vi "Example - Simple Move.vi"() -> ()   [LabVIEW 2017]
uses:
  SmartMotor_class/SmartMotor.lvclass
panel:
  in  "Start Motor 3":bool
  in  "Stop Motor 3":bool
  in  "Reset Motor Faults":bool
  in  "Start Motor 2":bool
  in  "Stop Motor 2":bool
  in  "SmartMotor Chain VISA Resource":refnum<visa-resource-name>="COM12"
  in  "Number of Motors In Motor Chain":i32=6 min=0 max=10 step=1
  in  "Start Motor":bool
  in  "Stop Motor":bool
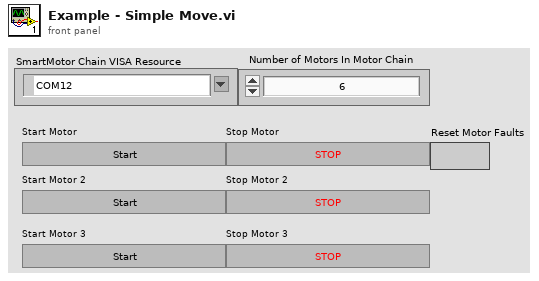
[diagram p1: front panel]
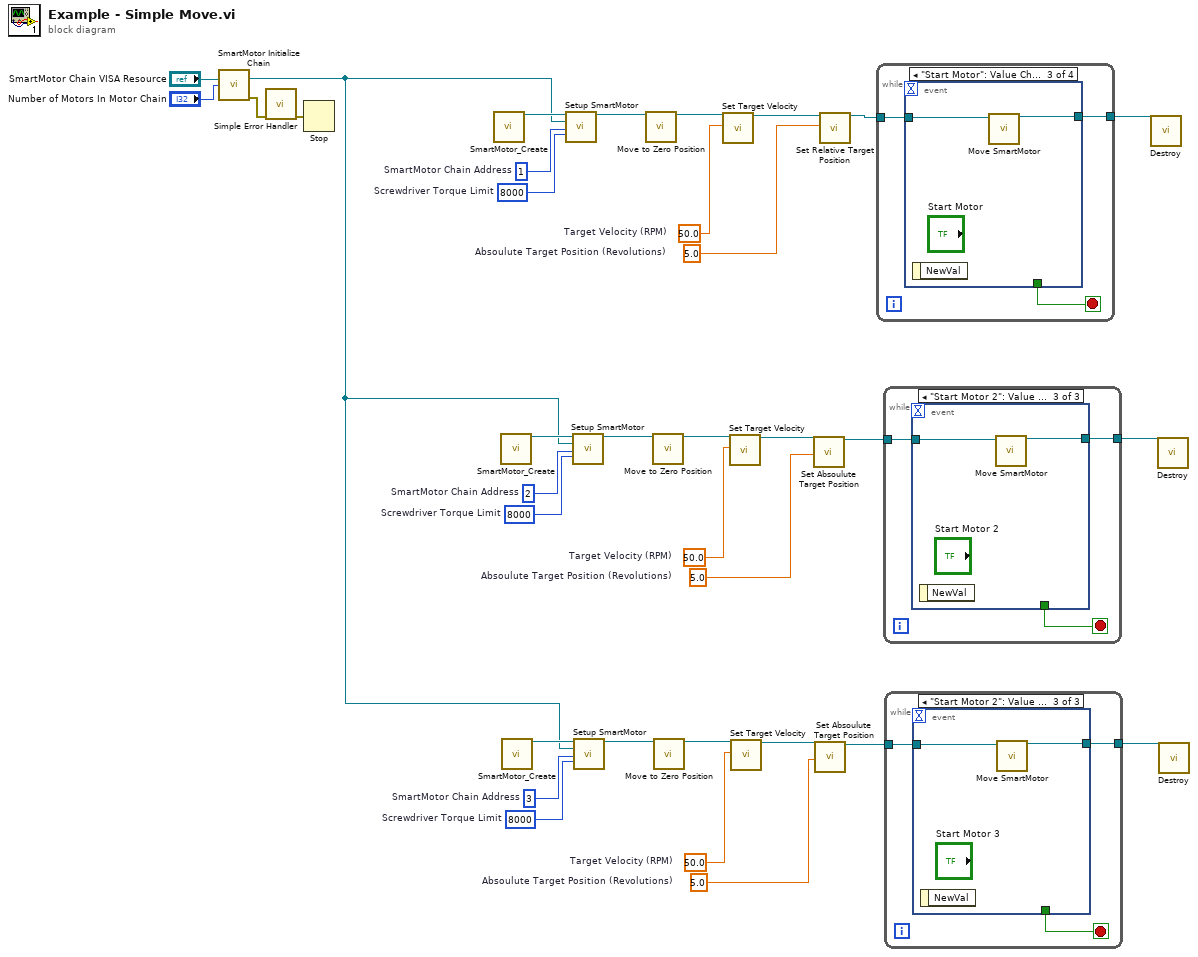
[diagram p0: block diagram]
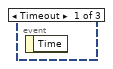
[diagram p2: hidden frame]
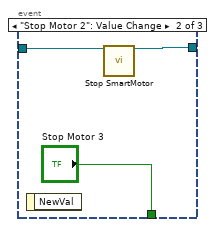
[diagram p3: hidden frame]
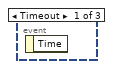
[diagram p4: hidden frame]
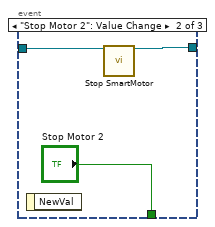
[diagram p5: hidden frame]
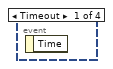
[diagram p6: hidden frame]
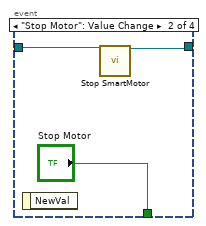
[diagram p7: hidden frame]
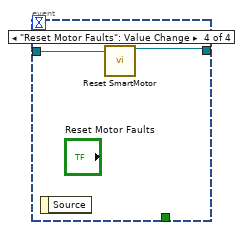
[diagram p8: hidden frame]
diagram:
  w11 = 5.0  # Absoulute Target Position (Revolutions)
  w10 = 50.0  # Target Velocity (RPM)
  w4 = 8000  # Screwdriver Torque Limit
  w3 = 3  # SmartMotor Chain Address
  w16 = 5.0  # Absoulute Target Position (Revolutions)
  w17 = 50.0  # Target Velocity (RPM)
  w23 = 8000  # Screwdriver Torque Limit
  w24 = 2  # SmartMotor Chain Address
  w12 = 5.0  # Absoulute Target Position (Revolutions)
  w27 = 50.0  # Target Velocity (RPM)
  w33 = 8000  # Screwdriver Torque Limit
  w34 = 1  # SmartMotor Chain Address
  n1 = call "SmartMotor Initialize Chain.vi"("SmartMotor Chain VISA Resource"="SmartMotor Chain VISA Resource", "Number of Motors In Motor Chain"="Number of Motors In Motor Chain") -> ("SmartMotor Chain VISA Session"=w1:refnum<visa-resource-name>, "Error Out"=w15:errorcluster)  [unwired: 11 in, 1 out]
  n2 = call <vilib>:"Simple Error Handler.vi"("error in (no error)"=w15) -> ("error out"=w26:errorcluster)  [unwired: 4 in, 4 out]
  n3 = Stop(stop? (T)=w26) -> ()
  n4 = call "SmartMotor_Create.vi"() -> ("reference out"=w32:refnum<class "SmartMotor.lvclass">)  [unwired: 18 in, 1 out]
  n5 = call "SmartMotor_Create.vi"() -> ("reference out"=w22:refnum<class "SmartMotor.lvclass">)  [unwired: 18 in, 1 out]
  n6 = call "SmartMotor_Create.vi"() -> ("reference out"=w5:refnum<class "SmartMotor.lvclass">)  [unwired: 18 in, 1 out]
  n7 = call-dynamic "Setup SmartMotor.vi"("reference in"=w32, "SmartMotor Chain VISA Session"=w1, "SmartMotor Chain Address"=w34, "Screwdriver Torque Limit"=w33) -> ("reference out"=w35:refnum<class "SmartMotor.lvclass">)  [unwired: 13 in, 2 out]
  n8 = call-dynamic "Setup SmartMotor.vi"("reference in"=w22, "SmartMotor Chain VISA Session"=w1, "SmartMotor Chain Address"=w24, "Screwdriver Torque Limit"=w23) -> ("reference out"=w25:refnum<class "SmartMotor.lvclass">)  [unwired: 13 in, 2 out]
  n9 = call-dynamic "Setup SmartMotor.vi"("reference in"=w5, "SmartMotor Chain VISA Session"=w1, "SmartMotor Chain Address"=w3, "Screwdriver Torque Limit"=w4) -> ("reference out"=w2:refnum<class "SmartMotor.lvclass">)  [unwired: 13 in, 2 out]
  n10 = call-dynamic "Move to Zero Position.vi"("reference in"=w35) -> ("reference out"=w31:refnum<class "SmartMotor.lvclass">)  [unwired: 17 in, 1 out]
  n11 = call-dynamic "Move to Zero Position.vi"("reference in"=w25) -> ("reference out"=w21:refnum<class "SmartMotor.lvclass">)  [unwired: 17 in, 1 out]
  n12 = call-dynamic "Move to Zero Position.vi"("reference in"=w2) -> ("reference out"=w6:refnum<class "SmartMotor.lvclass">)  [unwired: 17 in, 1 out]
  n13 = call-dynamic "Set Target Velocity.vi"("reference in"=w31, "Target Velocity (RPM)"=w27) -> ("reference out"=w13:refnum<class "SmartMotor.lvclass">)  [unwired: 16 in, 1 out]
  n14 = call-dynamic "Set Target Velocity.vi"("reference in"=w21, "Target Velocity (RPM)"=w17) -> ("reference out"=w20:refnum<class "SmartMotor.lvclass">)  [unwired: 16 in, 1 out]
  n15 = call-dynamic "Set Target Velocity.vi"("reference in"=w6, "Target Velocity (RPM)"=w10) -> ("reference out"=w7:refnum<class "SmartMotor.lvclass">)  [unwired: 16 in, 1 out]
  n16 = call-dynamic "Set Absoulute Target Position.vi"("reference in"=w20, "Absoulute Target Position (Revolutions)"=w16) -> ("reference out"=w19:refnum<class "SmartMotor.lvclass">)  [unwired: 16 in, 1 out]
  n17 = call-dynamic "Set Absoulute Target Position.vi"("reference in"=w7, "Absoulute Target Position (Revolutions)"=w11) -> ("reference out"=w8:refnum<class "SmartMotor.lvclass">)  [unwired: 16 in, 1 out]
  n18 = call-dynamic "Set Relative Target Position.vi"("reference in"=w13, "Relative Target Position (Revolutions)"=w12) -> ("reference out"=w14:refnum<class "SmartMotor.lvclass">)  [unwired: 16 in, 1 out]
  n19 = while {
    tunnel: w14 -> [w37]
    tunnel: [w36] -> w30
    stop <- w38 stop-if-true
    n20 = event shown="[2] \"Start Motor\": Value Change" {
      selector: _ -> [_ _ _ _]
      dyn-events: _ -> [_ _ _ _]
      timeout: _ -> [_ _ _ _]
      tunnel: [_ "Stop Motor" _ _] -> w38
      tunnel: w37 -> [_ w40 w43 w45]
      tunnel: [_ w39 w42 w44] -> w36
      event Timeout {
        n21 = event-data() -> ()  [unwired: 1 in, 1 out]
      }
      event "Stop Motor": Value Change {
        n22 = event-data() -> ()  [unwired: 1 in, 1 out]
        n23 = call-dynamic "Stop SmartMotor.vi"("reference in"=w40) -> ("reference out"=w39:refnum<class "SmartMotor.lvclass">)  [unwired: 17 in, 1 out]
      }
      event "Start Motor": Value Change {
        n24 = event-data() -> ()  [unwired: 1 in, 1 out]
        n25 = call-dynamic "Move SmartMotor.vi"("reference in"=w43) -> ("reference out"=w42:refnum<class "SmartMotor.lvclass">)  [unwired: 17 in, 1 out]
      }
      event "Reset Motor Faults": Value Change {
        n26 = event-data() -> ()  [unwired: 1 in, 1 out]
        n27 = call-dynamic "Reset SmartMotor.vi"("reference in"=w45) -> ("reference out"=w44:refnum<class "SmartMotor.lvclass">)  [unwired: 17 in, 1 out]
      }
    }
  }
  n28 = while {
    tunnel: w19 -> [w47]
    tunnel: [w46] -> w18
    stop <- w48 stop-if-true
    n29 = event shown="[2] \"Start Motor 2\": Value Change" {
      selector: _ -> [_ _ _]
      dyn-events: _ -> [_ _ _]
      timeout: _ -> [_ _ _]
      tunnel: [_ "Stop Motor 2" _] -> w48
      tunnel: w47 -> [_ w50 w53]
      tunnel: [_ w49 w52] -> w46
      event Timeout {
        n30 = event-data() -> ()  [unwired: 1 in, 1 out]
      }
      event "Stop Motor 2": Value Change {
        n31 = event-data() -> ()  [unwired: 1 in, 1 out]
        n32 = call-dynamic "Stop SmartMotor.vi"("reference in"=w50) -> ("reference out"=w49:refnum<class "SmartMotor.lvclass">)  [unwired: 17 in, 1 out]
      }
      event "Start Motor 2": Value Change {
        n33 = event-data() -> ()  [unwired: 1 in, 1 out]
        n34 = call-dynamic "Move SmartMotor.vi"("reference in"=w53) -> ("reference out"=w52:refnum<class "SmartMotor.lvclass">)  [unwired: 17 in, 1 out]
      }
    }
  }
  n35 = while {
    tunnel: w8 -> [w55]
    tunnel: [w54] -> w9
    stop <- w56 stop-if-true
    n36 = event shown="[2] \"Start Motor 2\": Value Change" {
      selector: _ -> [_ _ _]
      dyn-events: _ -> [_ _ _]
      timeout: _ -> [_ _ _]
      tunnel: [_ "Stop Motor 3" _] -> w56
      tunnel: w55 -> [_ w58 w61]
      tunnel: [_ w57 w60] -> w54
      event Timeout {
        n37 = event-data() -> ()  [unwired: 1 in, 1 out]
      }
      event "Stop Motor 2": Value Change {
        n38 = event-data() -> ()  [unwired: 1 in, 1 out]
        n39 = call-dynamic "Stop SmartMotor.vi"("reference in"=w58) -> ("reference out"=w57:refnum<class "SmartMotor.lvclass">)  [unwired: 17 in, 1 out]
      }
      event "Start Motor 2": Value Change {
        n40 = event-data() -> ()  [unwired: 1 in, 1 out]
        n41 = call-dynamic "Move SmartMotor.vi"("reference in"=w61) -> ("reference out"=w60:refnum<class "SmartMotor.lvclass">)  [unwired: 17 in, 1 out]
      }
    }
  }
  n42 = call-dynamic "Destroy.vi"("reference in"=w30) -> ()  [unwired: 17 in, 2 out]
  n43 = call-dynamic "Destroy.vi"("reference in"=w18) -> ()  [unwired: 17 in, 2 out]
  n44 = call-dynamic "Destroy.vi"("reference in"=w9) -> ()  [unwired: 17 in, 2 out]
